vi "Node - Set ID.vi"(8 "error in (no error)":errorcluster, 11 "Node Configuration Properties In":T1) -> (0 "error out":errorcluster, 2 "Node Data Out":T6, 3 "Node Configuration Properties Out":T1)   [LabVIEW 2016, in "PXImc Router.lvlib"]
uses:
  PXImc Router.lvlib
  Controls/Node - Configuration.ctl
  Controls/Node/Local Node Properties.ctl
  Controls/Node/Node Ch Properties.ctl
  Controls/Data Type.ctl
  Controls/Node/Remote Node Properties.ctl
  Controls/Node Data.ctl
  <vilib>/NI Veristand/VeriStand Data/Byte Buffer/Byte Buffer.lvclass
  Controls/Node/Node - PXImc Parameters.ctl
  Controls/Node/Node - Writer Data.ctl
  Controls/Node/Node - Readers Data.ctl
  Controls/Node/Node - Reader Data.ctl
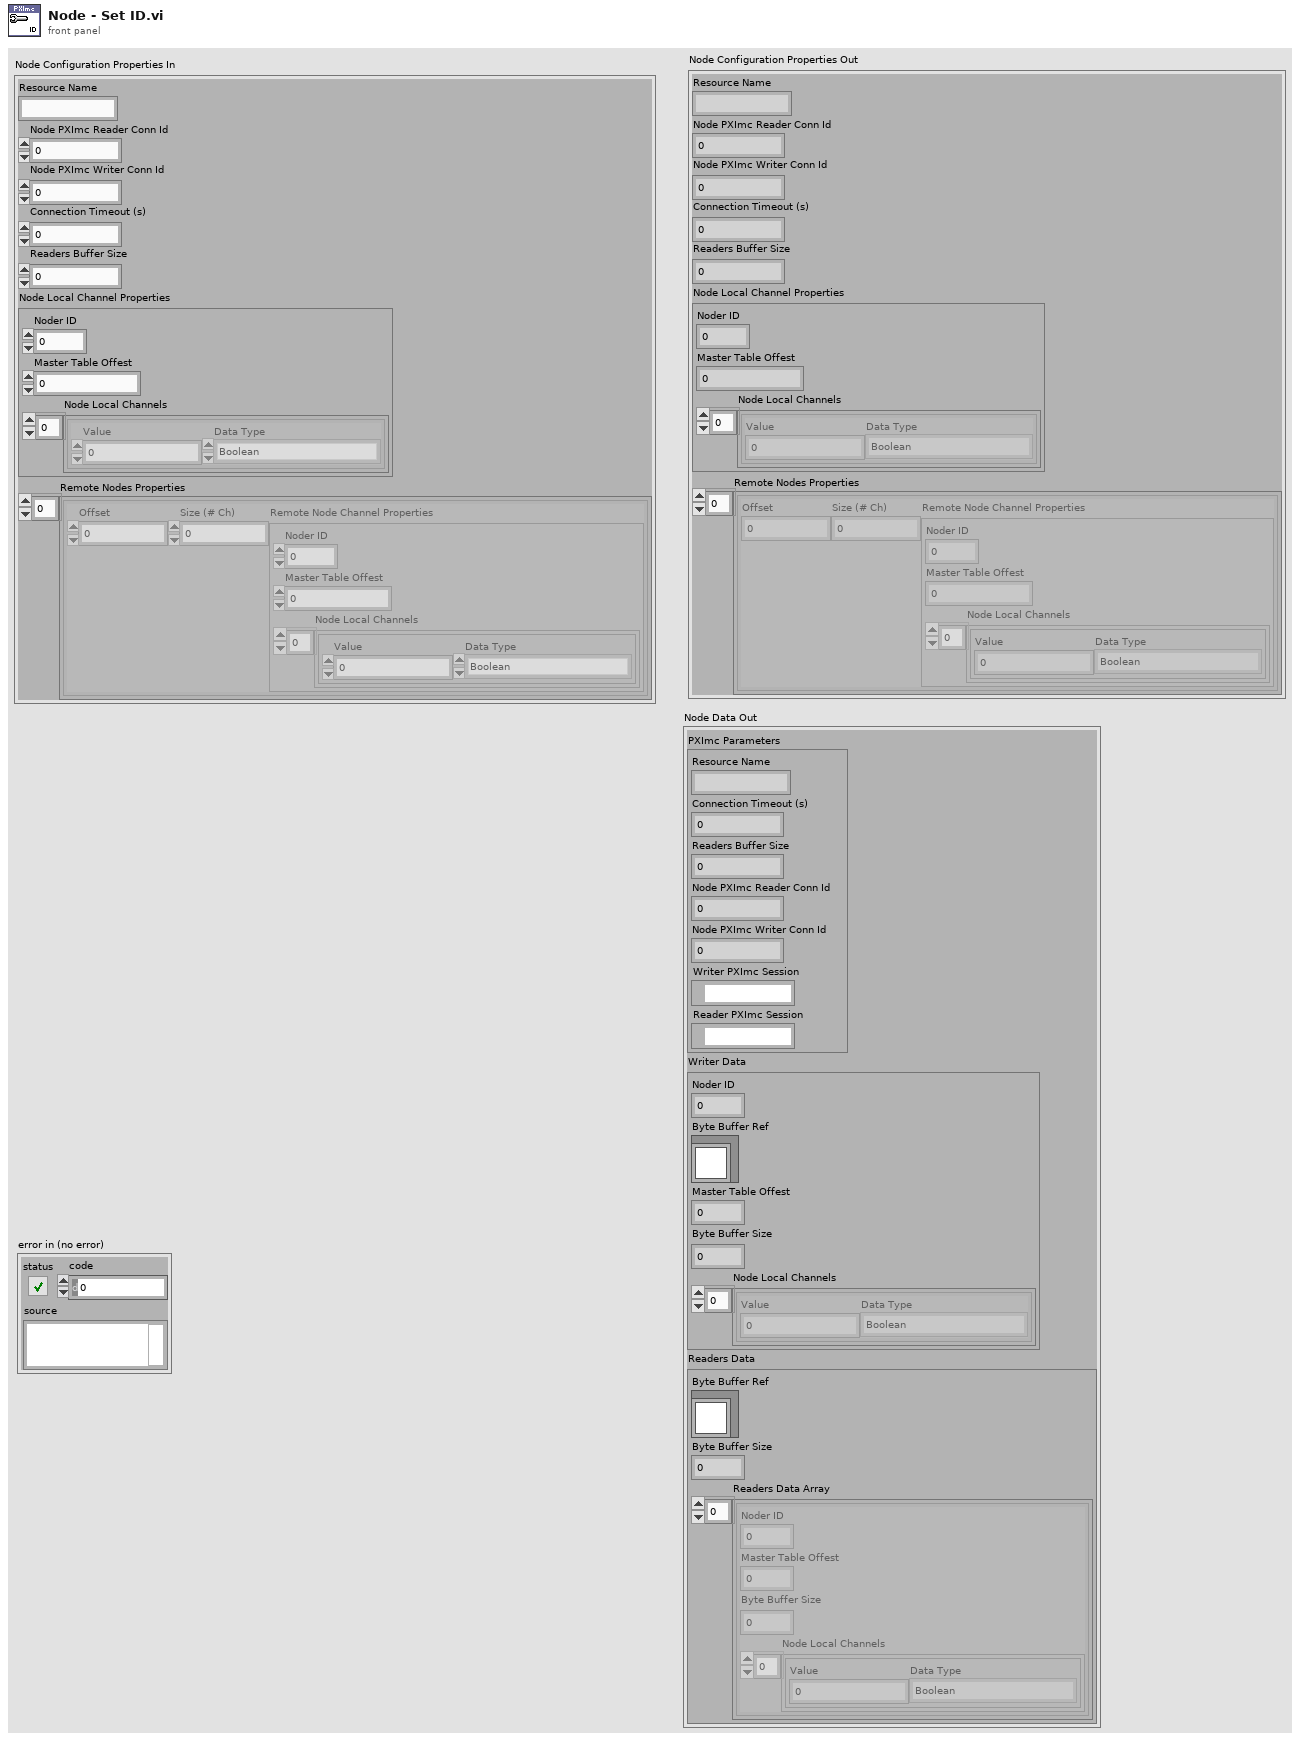
[diagram p1: front panel]
types:
  T1 = typedef "PXImc Router.lvlib/Node - Configuration.ctl" = cluster{"Resource Name":string, "Node PXImc Reader Conn Id":u16, "Node PXImc Writer Conn Id":u16, "Connection Timeout (s)":dbl, "Readers Buffer Size":u32, "Node Local Channel Properties":T2, "Remote Nodes Properties":T5[]}
  T2 = typedef "PXImc Router.lvlib/Local Node Properties.ctl" = cluster{"Noder ID":u32, "Master Table Offest":u32, "Node Local Channels":T3[]}
  T3 = typedef "PXImc Router.lvlib/Node Ch Properties.ctl" = cluster{"Value":dbl, "Data Type":T4}
  T4 = typedef "PXImc Router.lvlib/Data Type.ctl" = enum16{"Boolean", "SGL", "DBL", "I8", "I16", "I32", "I64", "U8", "U16", "U32", "U64"}
  T5 = typedef "PXImc Router.lvlib/Remote Node Properties.ctl" = cluster{"Offset":u32, "Size (# Ch)":u32, "Remote Node Channel Properties":T2}
  T6 = typedef "PXImc Router.lvlib/Node Data.ctl" = cluster{"PXImc Parameters":T7, "Writer Data":T8, "Readers Data":T9}
  T7 = typedef "PXImc Router.lvlib/Node - PXImc Parameters.ctl" = cluster{"Resource Name":string, "Connection Timeout (s)":dbl, "Readers Buffer Size":u64, "Node PXImc Reader Conn Id":u16, "Node PXImc Writer Conn Id":u16, "Writer PXImc Session":refnum<k21>, "Reader PXImc Session":refnum<k21>}
  T8 = typedef "PXImc Router.lvlib/Node - Writer Data.ctl" = cluster{"Noder ID":u32, "Byte Buffer Ref":refnum<class "Byte Buffer.lvclass">, "Master Table Offest":u32, "Byte Buffer Size":u32, "Node Local Channels":T3[]}
  T9 = typedef "PXImc Router.lvlib/Node - Readers Data.ctl" = cluster{"Byte Buffer Ref":refnum<class "Byte Buffer.lvclass">, "Byte Buffer Size":u64, "Readers Data Array":T10[]}
  T10 = typedef "PXImc Router.lvlib/Node - Reader Data.ctl" = cluster{"Noder ID":u32, "Master Table Offest":u32, "Byte Buffer Size":u64, "Node Local Channels":T3[]}
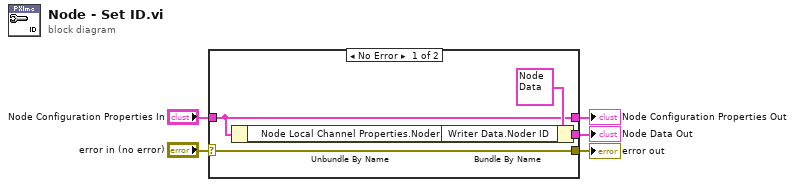
[diagram p0: block diagram]
diagram:
  n1 = case shown="No Error" "error in (no error)" {
    selector: "error in (no error)" -> [w10 w12]
    tunnel: [w10 w12] -> w4
    tunnel: "Node Configuration Properties In" -> [w6 w11]
    tunnel: [w7 _] -> w2
    tunnel: [w6 w11] -> w1
    frame No Error {
      n2 = Unbundle By Name(w6) -> ("Node Local Channel Properties.Noder ID"=w8:u32)
      n3 = Bundle By Name(cluster=T6 {"PXImc Parameters"={"Resource Name"="", "Connection Timeout (s)"=0.0, "Readers Buffer Size"=0, "Node PXImc Reader Conn Id"=0, "Node PXImc Writer Conn Id"=0, "Writer PXImc Session"="", "Reader PXImc Session"=""}, "Writer Data"={"Noder ID"=0, "Byte Buffer Ref"=refnum, "Master Table Offest"=0, "Byte Buffer Size"=0, "Node Local Channels"=[]}, "Readers Data"={"Byte Buffer Ref"=refnum, "Byte Buffer Size"=0, "Readers Data Array"=[]}} ("Node Data Out"), "Writer Data.Noder ID"=w8) -> (w7:T6)
    }
    frame Error {
    }
  }
  "error out" <- w4
  "Node Data Out" <- w2
  "Node Configuration Properties Out" <- w1
